vi "Terminate Vi CallStack Chain.vi"(7 "VI Refnum(Null)":refnum<vi>, 10 "ms timeout (500ms)":i32=500, 11 "Kill Process?":bool) -> ()   [LabVIEW 2017]
doc: "Waits for the call chain of VI Refnum(Null) to finish and then either stops it or kills the process, depending on Kill Process?. The ms timeout (500ms) input bounds the wait."
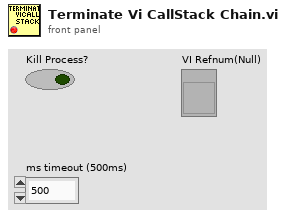
[diagram p1: front panel]
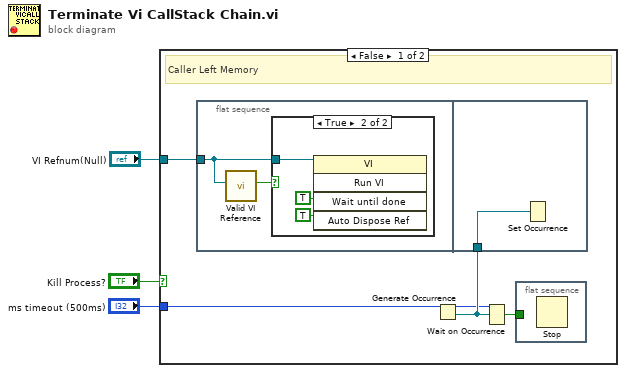
[diagram p0: block diagram]
diagram:
  n1 = case shown="False" "Kill Process?" {
    tunnel: "ms timeout (500ms)" -> [w5 _]
    tunnel: "VI Refnum(Null)" -> [w4 _]
    frame False {
      # "Caller Left Memory"
      n2 = flat-sequence {
        tunnel: w4 -> [w8]
        tunnel: w6 -> [w13]
        frame #0 {
          n3 = call "Valid VI Reference.vi"("VI Refnum"=w8) -> ("Valid?"=w9:bool)  [unwired: 9 in]
          n4 = case shown="True" w9 {
            tunnel: w8 -> [_ w12]
            frame False {
            }
            frame True {
              n5 = invoke class="VI" method="Run VI"(reference=w12, "Wait until done"=TRUE ("Wait Until Done"), "Auto Dispose Ref"=TRUE ("Auto Dispose Reference")) -> ()  [unwired: 2 in, 5 out]
            }
          }
        }
        frame #1 {
          n6 = Set Occurrence(w13) -> ()
        }
      }
      n7 = Generate Occurrence() -> (w6:refnum<k4>)
      n8 = Wait on Occurrence(2:w6, 3:w5) -> (0:w7:bool)  [unwired: 1 in]
      n9 = flat-sequence {
        tunnel: w7 -> [_]
        frame #0 {
          n10 = Stop() -> ()  [unwired: 1 in]
        }
      }
    }
    frame True {
      # "Process Terminated Normally"
    }
  }
